vi "Main.vi"(11 "Module Admin":refnum<class "Delacor_lib_QMH_Cloneable Module Admin.lvclass">) -> ()   [LabVIEW 2020, in "Cloneable Module.lvlib"]
doc: "This template is based off of the Queued Message Handler design pattern and the Queued Message Handler project template that ships with LabVIEW.\n\nThe main difference is that the queue is private to this module and communication between modules is performed via Broadcast and Request events.\n\nRequest events are wrapped in public API methods and are handled in the Event Handling Loop (EHL) of this VI. Any module can register for Broadcast events sent by this module. The EHL generates messages based on user interface actions.\n\nThe Message Handling Loop (MHL) processes messages generated by the EHL, or by other messages. The messages are string values, so new messages can be added easily to the Message Cases case structure in the MHL. Each message cluster can also provide an optional value for Message Data, which is a variant that can be converted to whatever message-specific data is required.\n_____\nBased on DQMH Project Template 6.1.0.93."
uses:
  Cloneable Module.lvlib
  <vilib>/Delacor/Delacor QMH/Libraries/Message Queue_class/Delacor_lib_QMH_Message Queue.lvclass
  Module Data--cluster.ctl
  <vilib>/Utility/miscctls.llb/LVPointTypeDef.ctl
  Do Something Argument--cluster.ctl
  Do Something Else Argument--cluster.ctl
  Do Something Else and Wait (Reply Payload)--cluster.ctl
  Do Something Else and Wait for Reply Argument--cluster.ctl
  <vilib>/Utility/error.llb/Error Cluster From Error Code.vi
  <vilib>/ErrorRing/Error Ring.xnode
  <vilib>/Delacor/Delacor QMH/Libraries/Message Queue_class/Delacor_lib_QMH_Enqueue Message (Single).vi
  Stop Argument--cluster.ctl
  <vilib>/Delacor/Delacor QMH/Libraries/Cloneable Module Admin_class/Delacor_lib_QMH_Cloneable Module Admin.lvclass
  ADD (Reply Payload)--cluster.ctl
  ADD Argument--cluster.ctl
panel:
  out "error out":errorcluster
  out "X":dbl
  out "Status":string
  in  "Simulate EHL Error":bool
  in  "Simulate MHL Error":bool
  in  "Do Something Else <Replace Me>":bool
  in  "Do Something <Replace Me>":bool
  # "These controls have associated \"Value Changed\" events configured in the Event Structure on the diagram.\n\nReplace them (and reconfigure the Event Structure) with the controls you need for your application. \n\nOther QMH Modules communicate with this Module via its Public API (wrappers for its Request Events).\n\nThis Module communicates with other Modules via its Broadcast Events.\nAny module that wants to get these messages, just registers for this module's Broadcast events."
  # "This template is for the Delacor Modified Queued Message Handler design pattern.\n\nSee the block diagram for more information on how to use this template."
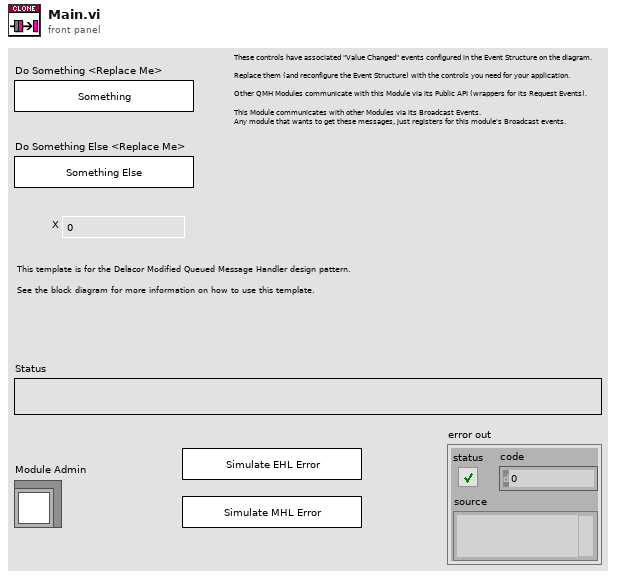
[diagram p1: front panel]
types:
  T1 = typedef "Cloneable Module.lvlib/Request Events--cluster.ctl" = cluster{"Stop Module":refnum<user-event>, "Do Something":refnum<user-event>, "Do Something Else":refnum<user-event>, "Do Something Else and Wait for Reply":refnum<user-event>, "Show Panel":refnum<user-event>, "Hide Panel":refnum<user-event>, "Show Diagram":refnum<user-event>, "Get Module Execution Status":refnum<user-event>, "ADD":refnum<user-event>}
  T2 = typedef "Cloneable Module.lvlib/Module Data--cluster.ctl" = cluster{"Status":string}
  T3 = typedef "Cloneable Module.lvlib/Do Something Argument--cluster.ctl" = cluster{"Module ID":i32, "Do Something Msg":string}
  T4 = typedef "Cloneable Module.lvlib/Do Something Else Argument--cluster.ctl" = cluster{"Module ID":i32, "Do Something Else Msg":string, "X":dbl}
  T5 = typedef "Cloneable Module.lvlib/Do Something Else and Wait for Reply Argument--cluster.ctl" = cluster{"Module ID":i32, "Do Something Else Msg":string, "X":dbl, "Wait Notifier":refnum<notifier>, "wait for reply":bool}
  T6 = enum32{"invalid lock state", "Not Locked", "Locked (No Password)", "Password-protected"}
  T7 = typedef "Cloneable Module.lvlib/Stop Argument--cluster.ctl" = cluster{"Module ID":i32, "Origin":string, "Exit via Stop Module Req?":bool, "Wait for Module to stop?":bool}
  T8 = typedef "Cloneable Module.lvlib/ADD Argument--cluster.ctl" = cluster{"Module ID":i32, "A":dbl, "B":dbl, "Wait Notifier":refnum<notifier>, "wait for reply":bool}
  T9 = typedef "LVPointTypeDef.ctl" = cluster{"Horizontal":i16, "Vertical":i16}
  T10 = enum32{"Invalid", "Standard", "Closed", "Hidden", "Minimized", "Maximized"}
  T11 = typedef "Cloneable Module.lvlib/Do Something Else and Wait (Reply Payload)--cluster.ctl" = cluster{"Value":dbl, "error":errorcluster}
  T12 = typedef "Cloneable Module.lvlib/ADD (Reply Payload)--cluster.ctl" = cluster{"A+B":dbl, "error":errorcluster}
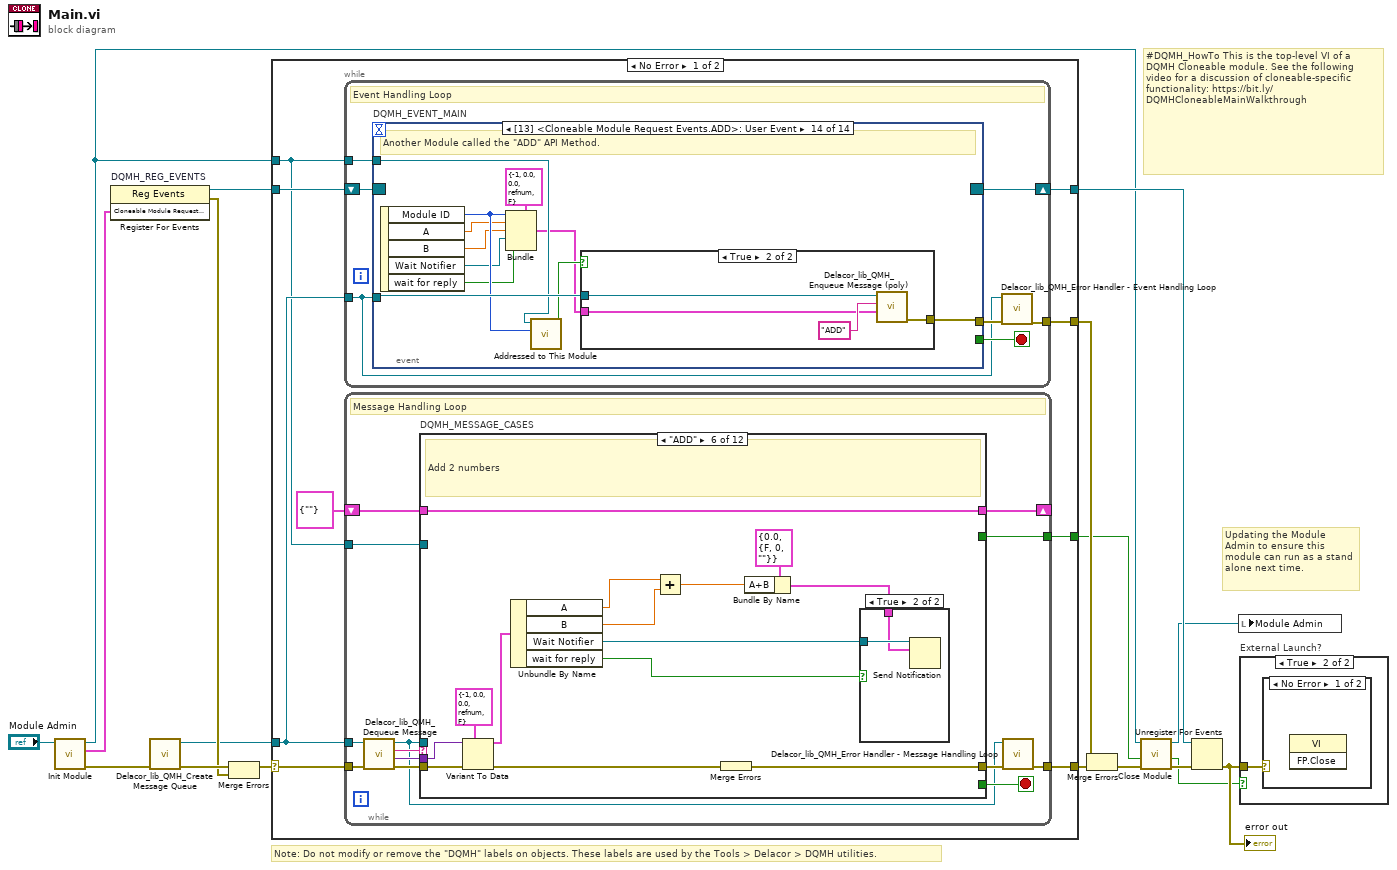
[diagram p0: block diagram]
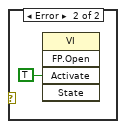
[diagram p3: hidden frame]
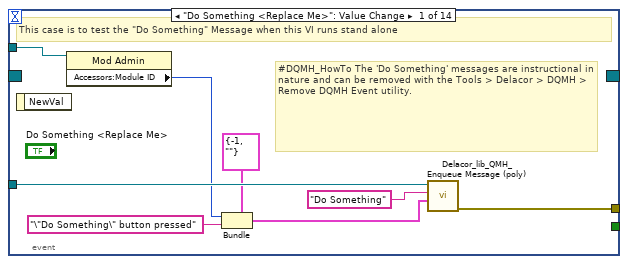
[diagram p4: hidden frame]
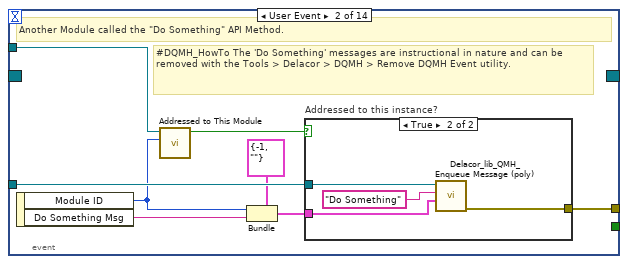
[diagram p5: hidden frame]
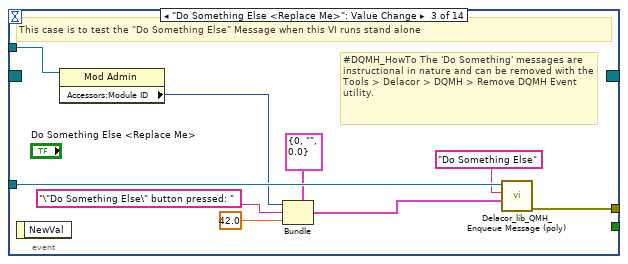
[diagram p7: hidden frame]
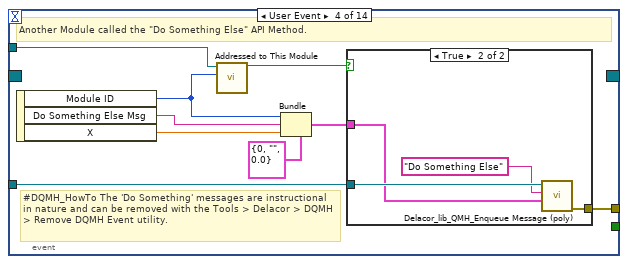
[diagram p8: hidden frame]
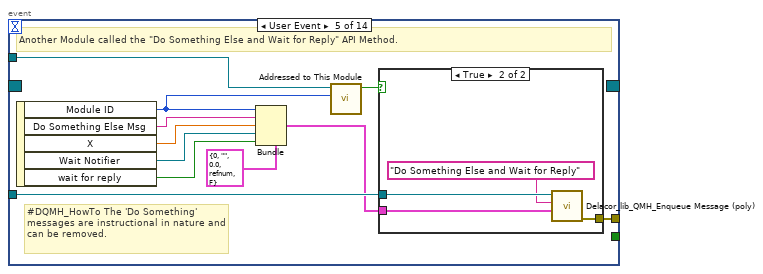
[diagram p10: hidden frame]
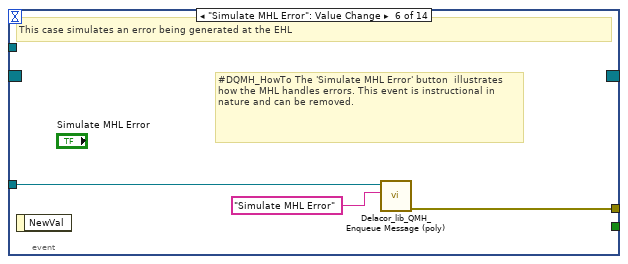
[diagram p12: hidden frame]
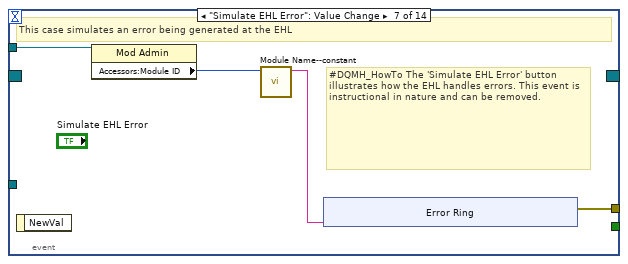
[diagram p13: hidden frame]
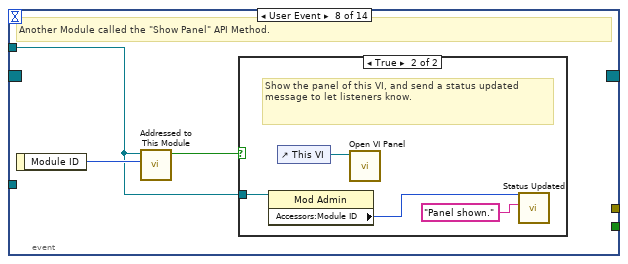
[diagram p14: hidden frame]
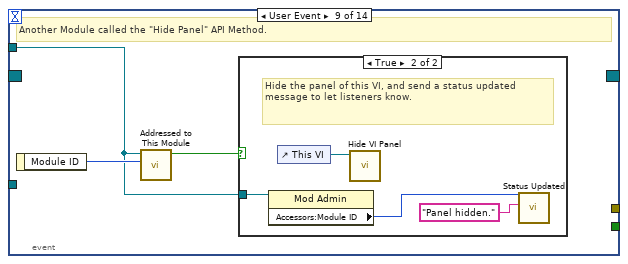
[diagram p16: hidden frame]
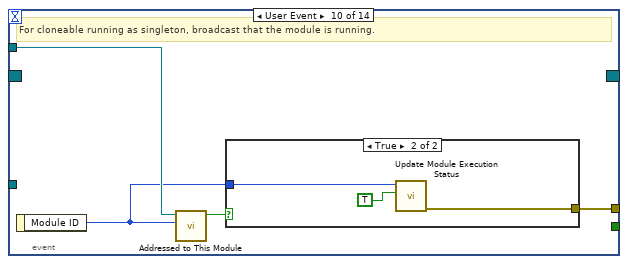
[diagram p18: hidden frame]
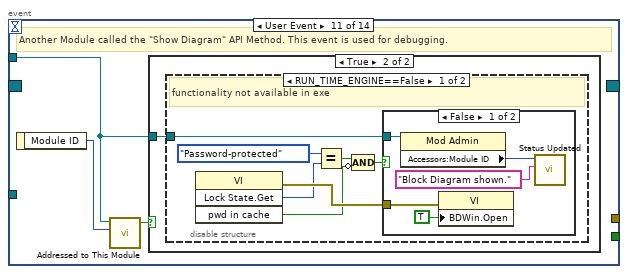
[diagram p20: hidden frame]
diagram:
  # "#DQMH_HowTo This is the top-level VI of a DQMH Cloneable module. See the following video for a discussion of cloneable-specific functionality: https://bit.ly/DQMHCloneableMainWalkthrough"
  # "Note: Do not modify or remove the \"DQMH\" labels on objects. These labels are used by the Tools > Delacor > DQMH utilities."
  # "Updating the Module Admin to ensure this module can run as a stand alone next time."
  n1 = call "Init Module.vi"("Cloneable Module Admin in"="Module Admin") -> ("error out"=w15:errorcluster, "Cloneable Module Request Events"=w7:T1, "Cloneable Module Admin out"=w4:refnum<class "Delacor_lib_QMH_Cloneable Module Admin.lvclass">)  [unwired: 8 in]
  n2 = register-events "DQMH_REG_EVENTS"(w7) -> (reference out=w8:refnum<event-registration>, error out=w10:errorcluster)  [unwired: 2 in]
  n3 = call <vilib>:"Delacor_lib_QMH_Create Message Queue.vi"("error in"=w15) -> ("error out"=w12:errorcluster, "Message Queue"=w6:refnum<class "Delacor_lib_QMH_Message Queue.lvclass">)  [unwired: 9 in]
  n4 = Merge Errors(w12, w10) -> (w11:errorcluster)
  n5 = case shown="No Error" w11 {
    selector: w11 -> [w25 w365]
    tunnel: [w27 w364] -> w16
    tunnel: [w24 w372] -> w9
    tunnel: w8 -> [w22 w372]
    tunnel: w6 -> [w21 w363]
    tunnel: [w26 _] -> w17
    tunnel: w4 -> [w20 w368]
    tunnel: [w19 _] -> w2
    frame No Error {
      n6 = while {
        tunnel: w21 -> [w28]
        shift-right: [w31] -> w24
        shift-left: w22 -> [w32]
        tunnel: [w33] -> w26
        tunnel: w20 -> [w29]
        stop <- w30 stop-if-true
        # "Event Handling Loop"
        n7 = event "DQMH_EVENT_MAIN" shown="[13] <Cloneable Module Request Events.ADD>: User Event" {
          selector: w32 -> [_ _ _ _ _ _ _ _ _ _ _ _ _ _]
          dyn-events: [_ _ _ _ _ _ _ _ _ _ _ _ _ _] -> w31
          timeout: _ -> [_ _ _ _ _ _ _ _ _ _ _ _ _ _]
          tunnel: [_ _ _ _ _ _ _ _ _ _ _ w146 _ _] -> w30
          tunnel: w28 -> [w41 w49 w62 w71 w86 w93 _ _ _ _ _ w149 w165 w184]
          tunnel: [w42 w50 w63 w72 w87 w94 w98 _ _ w123 _ w150 w168 w174] -> w34
          tunnel: w29 -> [w37 w47 w56 w69 w84 _ w97 w106 w113 w121 w127 w148 w166 w182]
          event "Do Something <Replace Me>": Value Change {
            # "#DQMH_HowTo The 'Do Something' messages are instructional in nature and can be removed with the Tools > Delacor > DQMH > Remove DQMH Event utility."
            # "This case is to test the \"Do Something\" Message when this VI runs stand alone"
            n8 = event-data() -> ()  [unwired: 1 in, 1 out]
            n9 = property class="Mod Admin"(reference=w37) -> ("Accessors:Module ID"=w36:i32)  [unwired: 1 in, 2 out]
            n10 = Bundle(cluster=T3 {"Module ID"=-1, "Do Something Msg"=""} ("Do Something Argument"), "Module ID"=w36, "Do Something Msg"="\"Do Something\" button pressed" ("\"Do Something\" button pressed")) -> (w39:T3)
            n11 = call-poly <vilib>:"Delacor_lib_QMH_Enqueue Message (poly).vi"("Message Data"=w39, "Message"="Do Something", "Message Queue in"=w41) -> ("error out"=w42:errorcluster)  [unwired: 7 in, 1 out]
          }
          event User Event {
            # "#DQMH_HowTo The 'Do Something' messages are instructional in nature and can be removed with the Tools > Delacor > DQMH > Remove DQMH Event utility."
            # "Another Module called the \"Do Something\" API Method."
            n12 = event-data() -> ("Module ID"=w44:i32, "Do Something Msg"=w43:string)  [unwired: 1 in]
            n13 = call "Addressed to This Module.vi"("Module ID from Argument"=w44, "Module Admin"=w47) -> ("Addressed to this instance?"=w48:bool)  [unwired: 8 in, 1 out]
            n14 = Bundle(cluster=T3 {"Module ID"=-1, "Do Something Msg"=""} ("Do Something Argument"), "Module ID"=w44, "Do Something Msg"=w43) -> (w46:T3)
            n15 = case "Addressed to this instance?" shown="True" w48 {
              tunnel: w49 -> [_ w53]
              tunnel: [_ w54] -> w50
              tunnel: w46 -> [_ w51]
              frame False {
                # "Do nothing"
              }
              frame True {
                n16 = call-poly <vilib>:"Delacor_lib_QMH_Enqueue Message (poly).vi"("Message Data"=w51, "Message"="Do Something", "Message Queue in"=w53) -> ("error out"=w54:errorcluster)  [unwired: 7 in, 1 out]
              }
            }
          }
          event "Do Something Else <Replace Me>": Value Change {
            # "#DQMH_HowTo The 'Do Something' messages are instructional in nature and can be removed with the Tools > Delacor > DQMH > Remove DQMH Event utility."
            # "This case is to test the \"Do Something Else\" Message when this VI runs stand alone"
            n17 = event-data() -> ()  [unwired: 1 in, 1 out]
            n18 = property class="Mod Admin"(reference=w56) -> ("Accessors:Module ID"=w55:i32)  [unwired: 1 in, 2 out]
            n19 = Bundle(cluster=T4 {"Module ID"=0, "Do Something Else Msg"="", "X"=0.0} ("Do Something Else Argument"), "Module ID"=w55, "Do Something Else Msg"="\"Do Something Else\" button pressed: " ("\"Do Something Else\" button pressed"), "X"=42.0) -> (w59:T4)
            n20 = call-poly <vilib>:"Delacor_lib_QMH_Enqueue Message (poly).vi"("Message Data"=w59, "Message"="Do Something Else", "Message Queue in"=w62) -> ("error out"=w63:errorcluster)  [unwired: 7 in, 1 out]
          }
          event User Event {
            # "#DQMH_HowTo The 'Do Something' messages are instructional in nature and can be removed with the Tools > Delacor > DQMH > Remove DQMH Event utility."
            # "Another Module called the \"Do Something Else\" API Method."
            n21 = event-data() -> ("Module ID"=w64:i32, "Do Something Else Msg"=w65:string, "X"=w67:dbl)  [unwired: 1 in]
            n22 = call "Addressed to This Module.vi"("Module ID from Argument"=w64, "Module Admin"=w69) -> ("Addressed to this instance?"=w70:bool)  [unwired: 8 in, 1 out]
            n23 = Bundle(cluster=T4 {"Module ID"=0, "Do Something Else Msg"="", "X"=0.0} ("Do Something Else Argument"), "Module ID"=w64, "Do Something Else Msg"=w65, "X"=w67) -> (w66:T4)
            n24 = case shown="True" w70 {
              tunnel: w71 -> [_ w75]
              tunnel: [_ w76] -> w72
              tunnel: w66 -> [_ w73]
              frame False {
              }
              frame True {
                n25 = call-poly <vilib>:"Delacor_lib_QMH_Enqueue Message (poly).vi"("Message Data"=w73, "Message"="Do Something Else", "Message Queue in"=w75) -> ("error out"=w76:errorcluster)  [unwired: 7 in, 1 out]
              }
            }
          }
          event User Event {
            # "#DQMH_HowTo The 'Do Something' messages are instructional in nature and can be removed."
            # "Another Module called the \"Do Something Else and Wait for Reply\" API Method."
            n26 = event-data() -> ("Module ID"=w82:i32, "Do Something Else Msg"=w80:string, "X"=w79:dbl, "Wait Notifier"=w78:refnum<notifier>, "wait for reply"=w77:bool)  [unwired: 1 in]
            n27 = Bundle(cluster=T5 {"Module ID"=0, "Do Something Else Msg"="", "X"=0.0, "Wait Notifier"=refnum, "wait for reply"=FALSE} ("Do Something Else and Wait for Reply Argument"), "Module ID"=w82, "Do Something Else Msg"=w80, "X"=w79, "Wait Notifier"=w78, "wait for reply"=w77) -> (w81:T5)
            n28 = call "Addressed to This Module.vi"("Module ID from Argument"=w82, "Module Admin"=w84) -> ("Addressed to this instance?"=w85:bool)  [unwired: 8 in, 1 out]
            n29 = case shown="True" w85 {
              tunnel: [_ w91] -> w87
              tunnel: w86 -> [_ w90]
              tunnel: w81 -> [_ w88]
              frame False {
              }
              frame True {
                n30 = call-poly <vilib>:"Delacor_lib_QMH_Enqueue Message (poly).vi"("Message Data"=w88, "Message"="Do Something Else and Wait for Reply", "Message Queue in"=w90) -> ("error out"=w91:errorcluster)  [unwired: 7 in, 1 out]
              }
            }
          }
          event "Simulate MHL Error": Value Change {
            # "#DQMH_HowTo The 'Simulate MHL Error' button  illustrates how the MHL handles errors. This event is instructional in nature and can be removed."
            # "This case simulates an error being generated at the EHL"
            n31 = event-data() -> ()  [unwired: 1 in, 1 out]
            n32 = call-poly <vilib>:"Delacor_lib_QMH_Enqueue Message (poly).vi"("Message"="Simulate MHL Error", "Message Queue in"=w93) -> ("error out"=w94:errorcluster)  [unwired: 8 in, 1 out]
          }
          event "Simulate EHL Error": Value Change {
            # "#DQMH_HowTo The 'Simulate EHL Error' button  illustrates how the EHL handles errors. This event is instructional in nature and can be removed."
            # "This case simulates an error being generated at the EHL"
            n33 = event-data() -> ()  [unwired: 1 in, 1 out]
            n34 = property class="Mod Admin"(reference=w97) -> ("Accessors:Module ID"=w96:i32)  [unwired: 1 in, 2 out]
            n35 = call "Module Name--constant.vi"("Module ID"=w96) -> ("Module Name"=w95:string)  [unwired: 10 in]
            n36 = xnode "Error Ring"("parameter 0"=w95) -> ("error out"=w98:errorcluster)
          }
          event User Event {
            # "Another Module called the \"Show Panel\" API Method."
            n37 = event-data() -> ("Module ID"=w107:i32)  [unwired: 1 in]
            n38 = call "Addressed to This Module.vi"("Module ID from Argument"=w107, "Module Admin"=w106) -> ("Addressed to this instance?"=w108:bool)  [unwired: 8 in, 1 out]
            n39 = case shown="True" w108 {
              tunnel: w106 -> [_ w110]
              frame False {
              }
              frame True {
                # "Show the panel of this VI, and send a status updated message to let listeners know."
                n40 = property class="Mod Admin"(reference=w110) -> ("Accessors:Module ID"=w109:i32)  [unwired: 1 in, 2 out]
                n41 = control-ref of="This VI"() -> (w112:refnum<vi>)
                n42 = call "Open VI Panel.vi"("VI"=w112) -> ()  [unwired: 10 in, 1 out]
                n43 = call "Status Updated.vi"("Status"="Panel shown." ("format string"), "Module ID"=w109) -> ()  [unwired: 9 in, 1 out]
              }
            }
          }
          event User Event {
            # "Another Module called the \"Hide Panel\" API Method."
            n44 = event-data() -> ("Module ID"=w114:i32)  [unwired: 1 in]
            n45 = call "Addressed to This Module.vi"("Module ID from Argument"=w114, "Module Admin"=w113) -> ("Addressed to this instance?"=w115:bool)  [unwired: 8 in, 1 out]
            n46 = case shown="True" w115 {
              tunnel: w113 -> [_ w117]
              frame False {
              }
              frame True {
                # "Hide the panel of this VI, and send a status updated message to let listeners know."
                n47 = property class="Mod Admin"(reference=w117) -> ("Accessors:Module ID"=w116:i32)  [unwired: 1 in, 2 out]
                n48 = control-ref of="This VI"() -> (w119:refnum<vi>)
                n49 = call "Hide VI Panel.vi"("VI"=w119) -> ()  [unwired: 10 in, 1 out]
                n50 = call "Status Updated.vi"("Status"="Panel hidden." ("format string"), "Module ID"=w116) -> ()  [unwired: 9 in, 1 out]
              }
            }
          }
          event User Event {
            # "For cloneable running as singleton, broadcast that the module is running."
            n51 = event-data() -> ("Module ID"=w120:i32)  [unwired: 1 in]
            n52 = call "Addressed to This Module.vi"("Module ID from Argument"=w120, "Module Admin"=w121) -> ("Addressed to this instance?"=w122:bool)  [unwired: 8 in, 1 out]
            n53 = case shown="True" w122 {
              tunnel: [_ w126] -> w123
              tunnel: w120 -> [_ w125]
              frame False {
              }
              frame True {
                n54 = call "Update Module Execution Status.vi"("Running?"=TRUE, "Module ID"=w125) -> ("error out"=w126:errorcluster)  [unwired: 9 in]
              }
            }
          }
          event User Event {
            # "Another Module called the \"Show Diagram\" API Method. This event is used for debugging."
            n55 = event-data() -> ("Module ID"=w128:i32)  [unwired: 1 in]
            n56 = call "Addressed to This Module.vi"("Module ID from Argument"=w128, "Module Admin"=w127) -> ("Addressed to this instance?"=w129:bool)  [unwired: 8 in, 1 out]
            n57 = case shown="True" w129 {
              tunnel: w127 -> [_ w130]
              frame False {
              }
              frame True {
                n58 = disable-structure shown="RUN_TIME_ENGINE==False" {
                  disable-tunnel: w130 -> [w131 _]
                  frame condition #0 (active) {
                    # "functionality not available in exe"
                    n59 = invoke class="VI" method="Lock State.Get"() -> (error out=w137:errorcluster, "Get Lock State"=w136:T6, "pwd in cache"=w133:bool)  [unwired: 4 in, 1 out]
                    n60 = Equal?(x=T6."Password-protected", y=w136) -> (x = y?=w134:bool)
                    n61 = Compound Arithmetic op=AND(w134, invert w133) -> (w132:bool)
                    n62 = case shown="False" w132 {
                      tunnel: w137 -> [w142 _]
                      tunnel: w131 -> [w139 _]
                      frame False {
                        n63 = property class="Mod Admin"(reference=w139) -> ("Accessors:Module ID"=w138:i32)  [unwired: 1 in, 2 out]
                        n64 = property class="VI"(error in=w142, "BDWin.Open"=TRUE ("Block Diagram Window:Open")) -> ()  [unwired: 1 in, 2 out]
                        n65 = call "Status Updated.vi"("Status"="Block Diagram shown." ("format string"), "Module ID"=w138) -> ()  [unwired: 9 in, 1 out]
                      }
                      frame True {
                        # "Password-protected VI, and the password is not in the cache. Do not show the diagram."
                      }
                    }
                  }
                  frame condition #1 {
                  }
                }
              }
            }
          }
          event User Event {
            # "Another Module called the \"Stop Module\" API Method  or the Message Handling Loop below."
            n66 = event-data() -> ("Module ID"=w144:i32, "Wait for Module to stop?"=w145:bool, "Origin"=w143:string)  [unwired: 1 in]
            n67 = call "Addressed to This Module.vi"("Module ID from Argument"=w144, "Module Admin"=w148) -> ("Addressed to this instance?"=w147:bool)  [unwired: 8 in, 1 out]
            n68 = case shown="True" w147 {
              tunnel: [_ w162] -> w150
              tunnel: w149 -> [_ w158]
              tunnel: [_ TRUE] -> w146
              tunnel: w145 -> [_ w153]
              tunnel: w144 -> [_ w155]
              tunnel: w143 -> [_ w151]
              frame False {
              }
              frame True {
                # "The event can get fired from the Exit message. The queue gets destroyed there. In this case, the Enqueue VI will return error 1. It is safe to ignore, because the module is already exiting."
                n69 = local write "Status"(w151) -> ()
                n70 = Bundle By Name(cluster=T7 {"Module ID"=-1, "Origin"="", "Exit via Stop Module Req?"=FALSE, "Wait for Module to stop?"=FALSE} ("Stop Argument"), "Module ID"=w155, "Exit via Stop Module Req?"=TRUE, "Wait for Module to stop?"=w153) -> (w152:T7)
                n71 = call-poly <vilib>:"Delacor_lib_QMH_Enqueue Message (poly).vi"("Priority Message? (F)"=TRUE, "Message Data"=w152, "Message"="Exit", "Message Queue in"=w158) -> ("error out"=w163:errorcluster)  [unwired: 6 in, 1 out]
                n72 = call <vilib>:"Clear Errors.vi"("error in (no error)"=w163, "specific error code to clear (0: all)"=1) -> ("error out"=w162:errorcluster)  [unwired: 4 in, 1 out]
              }
            }
          }
          event Panel Close? {
            w167 = TRUE  # Discard the event, the MHL is responsible for closing and stopping this VI.
            # "Hide the panel or send the 'Exit' message if the user clicks the 'X' on the module main VI panel."
            n73 = event-data() -> ()  [unwired: 1 in, 1 out]
            n74 = property class="Mod Admin"(reference=w166) -> ("Accessors:External Launch"=w164:bool)  [unwired: 1 in, 2 out]
            n75 = case shown="True" w164 {
              tunnel: w165 -> [_ w172]
              tunnel: [_ w173] -> w168
              frame True {
                # "If externally launched, clicking the 'X' hides the panel, but doesn't close it."
                n76 = control-ref of="This VI"() -> (w169:refnum<vi>)
                n77 = call "Hide VI Panel.vi"("VI"=w169) -> ()  [unwired: 10 in, 1 out]
              }
              frame False {
                # "If run as a stand-alone VI, clicking the panel 'X' stops the VI."
                n78 = call-poly <vilib>:"Delacor_lib_QMH_Enqueue Message (poly).vi"("Priority Message? (F)"=TRUE, "Message"="Exit", "Message Queue in"=w172) -> ("error out"=w173:errorcluster)  [unwired: 7 in, 1 out]
              }
            }
            n79 = event-data("Discard?"=w167) -> ()  [unwired: 1 in, 1 out]
          }
          event User Event {
            # "Another Module called the \"ADD\" API Method."
            n80 = event-data() -> ("Module ID"=w179:i32, "A"=w178:dbl, "B"=w177:dbl, "Wait Notifier"=w176:refnum<notifier>, "wait for reply"=w175:bool)  [unwired: 1 in]
            n81 = Bundle(cluster=T8 {"Module ID"=-1, "A"=0.0, "B"=0.0, "Wait Notifier"=refnum, "wait for reply"=FALSE} ("ADD Argument"), "Module ID"=w179, "A"=w178, "B"=w177, "Wait Notifier"=w176, "wait for reply"=w175) -> (w180:T8)
            n82 = call "Addressed to This Module.vi"("Module ID from Argument"=w179, "Module Admin"=w182) -> ("Addressed to this instance?"=w183:bool)  [unwired: 8 in, 1 out]
            n83 = case shown="True" w183 {
              tunnel: w184 -> [_ w188]
              tunnel: w180 -> [_ w186]
              tunnel: [_ w185] -> w174
              frame False {
              }
              frame True {
                n84 = call-poly <vilib>:"Delacor_lib_QMH_Enqueue Message (poly).vi"("Message Data"=w186, "Message"="ADD", "Message Queue in"=w188) -> ("error out"=w185:errorcluster)  [unwired: 7 in, 1 out]
              }
            }
          }
        }
        n85 = call-dynamic "Delacor_lib_QMH_Error Handler - Event Handling Loop.vi"("error in"=w34, "Message Queue in"=w28) -> ("dup error in"=w33:errorcluster)  [unwired: 8 in, 1 out]
      }
      n86 = while {
        tunnel: w21 -> [w192]
        shift-right: [w196] -> _
        shift-left: T2 {"Status"=""} ("Data Cluster") -> [w197]
        tunnel: w25 -> [w200]
        tunnel: [w198] -> w27
        tunnel: w20 -> [w190]
        tunnel: [w189] -> w19
        stop <- w195 stop-if-true
        # "Message Handling Loop"
        n87 = call-dynamic "Delacor_lib_QMH_Dequeue Message.vi"("error in"=w200, "Message Queue in"=w192) -> ("error out"=w199:errorcluster, "Message Data"=w193:variant, "Message"=w194:string, "Message Queue out"=w191:refnum<class "Delacor_lib_QMH_Message Queue.lvclass">)  [unwired: 6 in]
        n88 = case "DQMH_MESSAGE_CASES" shown="\"ADD\"" w194 {
          selector: w194 -> [_ _ _ _ _ _ _ _ _ _ _ w350]
          tunnel: w191 -> [_ _ _ _ _ _ _ _ w301 _ w340 _]
          tunnel: w199 -> [w220 w224 w234 w245 w266 w292 w297 w299 w310 w323 w346 w352]
          tunnel: [w218 w224 w232 w244 w265 w282 w296 w299 w306 w322 w343 w353] -> w201
          tunnel: w197 -> [w211 w223 w231 w243 w263 w291 w295 w298 w305 w320 w339 w351]
          tunnel: [w210 w223 w231 w243 w263 w291 w295 w298 w305 w320 w339 w351] -> w196
          tunnel: [_ _ _ _ _ _ _ _ _ _ w338 _] -> w195
          tunnel: w193 -> [_ _ w230 w240 w260 w289 _ _ w304 _ w336 _]
          tunnel: w190 -> [w205 _ w226 w236 w250 _ _ _ w303 w318 w332 w348]
          tunnel: [_ _ _ _ _ _ _ _ _ _ w334 _] -> w189
          frame "Initialize" {
            w202 = "Initial Message" ("Initial Message")
            # "#CodeNeeded - Initialize the appearance of the front panel."
            # "#CodeNeeded - Initialize your state data here."
            # "Initialize - Any operation that needs to be done before the module can receive messages. Synchronize Caller Events.vi will inform Start Module.vi that the module has launched and is ready to receive messages. Module Did Init.vi will broadcast that the module initialized."
            n89 = call "Synchronize Caller Events.vi"("error in (no error)"=w220, "Module Admin"=w205) -> ("error out"=w219:errorcluster, "Module Admin out"=w204:refnum<class "Delacor_lib_QMH_Cloneable Module Admin.lvclass">)  [unwired: 8 in]
            n90 = property class="Mod Admin"(reference=w204) -> ("Accessors:Module ID"=w207:i32, "Accessors:External Launch"=w206:bool)  [unwired: 1 in, 2 out]
            n91 = call "Module Name--constant.vi"("Module ID"=w207) -> ("Module Name"=w215:string)  [unwired: 10 in]
            n92 = property class="VI"("Front Panel.Title"=w215) -> (reference out=w217:refnum<vi>, error out=w222:errorcluster)  [unwired: 2 in]
            n93 = Select(t=T10."Hidden" ("State"), s=w206, f=T10."Standard" ("State")) -> (s? t:f=w212:T10)
            n94 = invoke class="VI" method="FP.Open"(reference=w217, error in=w222, "State"=w212) -> (reference out=w216:refnum<vi>, error out=w221:errorcluster)  [unwired: 2 in, 3 out]
            n95 = call "Module Name--constant.vi"("Module ID"=w207) -> ("Module Name"=w208:string)  [unwired: 10 in]
            n96 = Bundle By Name(cluster=w211, "Status"=w202) -> (w210:T2)
            n97 = invoke class="VI" method="FP.Center"(reference=w216, error in=w221) -> ()  [unwired: 1 in, 3 out]
            n98 = property on="Pane" class="Pane"("Origin"=T9 {"Horizontal"=0, "Vertical"=0}) -> ()  [unwired: 2 in, 2 out]
            n99 = call "Module Did Init.vi"("error in (no error)"=w219, "Initialized?"=TRUE, "Origin"=w208, "Module ID"=w207) -> ("error out"=w218:errorcluster)  [unwired: 7 in]
            "Status" <- w202
          }
          frame "---Module Specific---" {
            # "Separator -- The following cases handle messages specific to this Module."
          }
          frame "Do Something" {
            # "#DQMH_HowTo The 'Do Something' messages are instructional in nature and can be removed with the Tools > Delacor > DQMH > Remove DQMH Event utility."
            # "Do Something - Replace this message with functionality for your own application. Note that this message also fires the \"Did Something\" broadcast event."
            n100 = property class="Mod Admin"(reference=w226) -> ("Accessors:Module ID"=w225:i32)  [unwired: 1 in, 2 out]
            n101 = Variant To Data(error in=w234, type=T3 {"Module ID"=-1, "Do Something Msg"=""} ("Do Something Argument"), Variant=w230) -> (data=w229:T3, error out=w233:errorcluster)
            n102 = Unbundle By Name(w229) -> ("Do Something Msg"=w227:string)
            n103 = call "Status Updated.vi"("Status"=w227, "Module ID"=w225) -> ()  [unwired: 9 in, 1 out]
            n104 = local write "Status"(w227) -> ()
            n105 = call "Did Something.vi"("error in (no error)"=w233, "Did Something Msg"=w227, "Module ID"=w225) -> ("error out"=w232:errorcluster)  [unwired: 8 in]
          }
          frame "Do Something Else" {
            # "#DQMH_HowTo The 'Do Something' messages are instructional in nature and can be removed with the Tools > Delacor > DQMH > Remove DQMH Event utility."
            # "Do Something Else - Replace this message with functionality for your own application."
            n106 = Variant To Data(error in=w245, type=T4 {"Module ID"=0, "Do Something Else Msg"="", "X"=0.0} ("Do Something Else Argument"), Variant=w240) -> (data=w241:T4, error out=w244:errorcluster)
            n107 = Unbundle By Name(w241) -> ("Do Something Else Msg"=w239:string, "X"=w238:dbl)
            "X" <- w238
            n108 = property class="Mod Admin"(reference=w236) -> ("Accessors:Module ID"=w235:i32)  [unwired: 1 in, 2 out]
            n109 = Format Into String(initial string=w239, w238) -> (resulting string=w237:string)  [unwired: 2 in, 1 out]
            n110 = call "Status Updated.vi"("Status"=w237, "Module ID"=w235) -> ()  [unwired: 9 in, 1 out]
            n111 = local write "Status"(w237) -> ()
          }
          frame "Do Something Else and Wait for Reply" {
            w253 = "X(%.2f)+Offset(%.2f)=%.2f"  # status message format string
            # "#DQMH_HowTo The 'Do Something' messages are instructional in nature and can be removed."
            # "Send back X with a random offset"
            # "Do Something Else and Wait for Reply - Replace this message with functionality for your own application. Note that this message must fire a notifier to let callers know it has finished execution, and it returns an error if the 'Value' is negative."
            n112 = Variant To Data(error in=w266, type=T5 {"Module ID"=0, "Do Something Else Msg"="", "X"=0.0, "Wait Notifier"=refnum, "wait for reply"=FALSE} ("Do Something Else and Wait for Reply Argument"), Variant=w260) -> (data=w261:T5, error out=w247:errorcluster)
            n113 = Unbundle By Name(w261) -> ("Wait Notifier"=w258:refnum<notifier>, "Do Something Else Msg"=w259:string, "X"=w255:dbl, "wait for reply"=w246:bool)
            n114 = property class="Mod Admin"(reference=w250) -> ("Accessors:Module ID"=w249:i32)  [unwired: 1 in, 2 out]
            n115 = Random Number (0-1)() -> (number: 0 to 1=w254:dbl)
            n116 = local write "X"(w255) -> ()
            n117 = Add(x=w254, y=w255) -> (x+y=w248:dbl)
            n118 = Format Into String(format string=w253, initial string=w259, w255, w254, w248) -> (resulting string=w251:string)  [unwired: 1 in, 1 out]
            n119 = Less Than 0?(x=w248) -> (x < 0?=w252:bool)
            n120 = case shown="True" w252 {
              tunnel: [_ w273] -> w264
              frame False {
              }
              frame True {
                n121 = xnode "Error Ring"() -> ("error out"=w273:errorcluster)
              }
            }
            n122 = Bundle By Name(cluster=T11 {"Value"=0.0, "error"={"status"=FALSE, "code"=0, "source"=""}} ("notification"), "error"=w264, "Value"=w248) -> (w256:T11)
            n123 = local write "Status"(w251) -> ()
            n124 = call "Status Updated.vi"("Status"=w251, "Module ID"=w249) -> ()  [unwired: 9 in, 1 out]
            n125 = case shown="True" w246 {
              tunnel: w258 -> [_ w270]
              tunnel: w256 -> [_ w269]
              frame False {
              }
              frame True {
                # "Simulate an operation that requires a wait."
                n126 = Wait (ms)(milliseconds to wait=u32 1000) -> (millisecond timer value=w267:u32)
                n127 = flat-sequence {
                  tunnel: w270 -> [w272]
                  tunnel: w269 -> [w271]
                  tunnel: w267 -> [_]
                  frame #0 {
                    n128 = Send Notification(notification=w271, notifier=w272) -> ()  [unwired: 1 in, 2 out]
                  }
                }
              }
            }
            n129 = Merge Errors(w247, w264) -> (w265:errorcluster)
          }
          frame "ADD" {
            # "Add 2 numbers"
            n130 = Variant To Data(error in=w292, type=T8 {"Module ID"=-1, "A"=0.0, "B"=0.0, "Wait Notifier"=refnum, "wait for reply"=FALSE} ("ADD Argument"), Variant=w289) -> (data=w287:T8, error out=w290:errorcluster)
            n131 = Unbundle By Name(w287) -> ("A"=w280:dbl, "B"=w279:dbl, "Wait Notifier"=w286:refnum<notifier>, "wait for reply"=w285:bool)
            n132 = Add(x=w280, y=w279) -> (x+y=w281:dbl)
            n133 = Merge Errors(w290) -> (w282:errorcluster)
            n134 = Bundle By Name(cluster=T12 {"A+B"=0.0, "error"={"status"=FALSE, "code"=0, "source"=""}} ("ADD (Reply Payload)"), "A+B"=w281) -> (w284:T12)
            n135 = case shown="True" w285 {
              tunnel: w286 -> [_ w294]
              tunnel: w284 -> [_ w293]
              frame False {
              }
              frame True {
                n136 = Send Notification(notification=w293, notifier=w294) -> ()  [unwired: 1 in, 2 out]
              }
            }
          }
          frame "---Copy This Frame---" {
            # "Duplicate this frame when creating new messages.  Change this comment in the duplicated frame to describe this message."
            n137 = Merge Errors(w297) -> (w296:errorcluster)
          }
          frame "---Exit and Error Handling---" {
            # "Separator - the following cases handle errors and exit messages."
          }
          frame "Error" {
            # "#CodeRecommended - If you ever change the name of this \"Error\" message, you'll need to update the name in the Check Loop Error.vi as well."
            # "#CodeRecommended - If the module is running in standalone mode (External Launch = FALSE), this code will pop up an error dialog and call the 'Exit' message if an error occurs. Add more fine-grained error handling here."
            # "Error - Check the error message data and respond accordingly. This message is sent by the \"Error Handler\" VIs at the end of each loop in this application."
            n138 = property class="Mod Admin"(reference=w303) -> ("Accessors:External Launch"=w302:bool, "Accessors:Module ID"=w300:i32)  [unwired: 1 in, 2 out]
            n139 = Variant To Data(error in=w310, type=errorcluster {"status"=FALSE, "code"=0, "source"=""} ("error constant"), Variant=w304) -> (data=w311:errorcluster, error out=w308:errorcluster)
            n140 = call "Error Reported.vi"("Error"=w311, "Module ID"=w300) -> ()  [unwired: 9 in, 1 out]
            n141 = case shown="False" w302 {
              tunnel: [w316 _] -> w307
              tunnel: w301 -> [w314 _]
              tunnel: w311 -> [w315 _]
              frame False {
                # "If the module is running standalone, then pop up an error dialog and call the \"Exit\" message."
                n142 = call <vilib>:"Simple Error Handler.vi"("error in (no error)"=w315) -> ()  [unwired: 4 in, 5 out]
                n143 = call-poly <vilib>:"Delacor_lib_QMH_Enqueue Message (poly).vi"("Priority Message? (F)"=TRUE, "Message"="Exit", "Message Queue in"=w314) -> ("error out"=w316:errorcluster)  [unwired: 7 in, 1 out]
              }
              frame True {
                # "If the module was launched externally, calling the Error Reported broadcast VI is the only action performed by the \"Error\" message. The module's caller can then process the error appropriately."
              }
            }
            n144 = Merge Errors(w308, w307) -> (w306:errorcluster)
            n145 = local write "error out"(w306) -> ()
          }
          frame "Simulate MHL Error" {
            # "#DQMH_HowTo The 'Simulate MHL Error' button  illustrates how the MHL handles errors. This event is instructional in nature and can be removed."
            # "Simulate an error occurring at the MHL"
            n146 = property class="Mod Admin"(reference=w318) -> ("Accessors:Module ID"=w319:i32)  [unwired: 1 in, 2 out]
            n147 = call "Module Name--constant.vi"("Module ID"=w319) -> ("Module Name"=w317:string)  [unwired: 10 in]
            n148 = xnode "Error Ring"("parameter 0"=w317) -> ("error out"=w321:errorcluster)
            n149 = Merge Errors(w323, w321) -> (w322:errorcluster)
          }
          frame "Exit" {
            w337 = 91  # 91: not all Exit messages will have an argument
            w338 = TRUE  # Stop the VI
            # "Release the message queue reference"
            # "#CodeNeeded - Add any required cleanup code here."
            # "Exit - Exit the application."
            n150 = Variant To Data(error in=w346, type=T7 {"Module ID"=-1, "Origin"="", "Exit via Stop Module Req?"=FALSE, "Wait for Module to stop?"=FALSE} ("Stop Argument"), Variant=w336) -> (data=w333:T7, error out=w341:errorcluster)
            n151 = call <vilib>:"Clear Errors.vi"("error in (no error)"=w341, "specific error code to clear (0: all)"=w337) -> ("error out"=w345:errorcluster)  [unwired: 4 in, 1 out]
            n152 = control-ref of="This VI"() -> (w331:refnum<vi>)
            n153 = call-dynamic "Delacor_lib_QMH_Release Message Queue.vi"("error in"=w345, "Message Queue"=w340) -> ("error out"=w344:errorcluster)  [unwired: 9 in]
            n154 = call "Handle Exit.vi"("Stop Argument"=w333, "Module Admin in"=w332, "VI reference"=w331) -> ("error out"=w342:errorcluster, "Wait for Stop?"=w334:bool)  [unwired: 7 in]
            n155 = Merge Errors(w344, w342) -> (w343:errorcluster)
          }
          frame Default {
            # "'Default' case only runs if there is a message that isn't defined in any of the other cases.  Output a programming error."
            n156 = property class="Mod Admin"(reference=w348) -> ("Accessors:Module ID"=w347:i32)  [unwired: 1 in, 2 out]
            n157 = call "Module Name--constant.vi"("Module ID"=w347) -> ("Module Name"=w349:string)  [unwired: 10 in]
            n158 = xnode "Error Ring"("parameter 0"=w350, "parameter 1"=w349) -> ("error out"=w354:errorcluster)
            n159 = Merge Errors(w352, w354) -> (w353:errorcluster)
          }
        }
        n160 = call-dynamic "Delacor_lib_QMH_Error Handler - Message Handling Loop.vi"("error in"=w201, "Message Queue in"=w191) -> ("dup error in"=w198:errorcluster)  [unwired: 8 in, 1 out]
      }
    }
    frame Error {
      n161 = call "Synchronize Caller Events.vi"("Module Admin"=w368) -> ("Module Admin out"=w367:refnum<class "Delacor_lib_QMH_Cloneable Module Admin.lvclass">)  [unwired: 9 in, 1 out]
      n162 = property class="Mod Admin"(reference=w367) -> ("Accessors:Module ID"=w366:i32)  [unwired: 1 in, 2 out]
      n163 = call-dynamic "Delacor_lib_QMH_Release Message Queue.vi"("error in"=w365, "Message Queue"=w363) -> ("error out"=w364:errorcluster)  [unwired: 9 in]
      n164 = call "Module Name--constant.vi"("Module ID"=w366) -> ("Module Name"=w371:string)  [unwired: 10 in]
      n165 = Format Into String(format string="An error occurred during initialization. %s is no longer running.", w371) -> (resulting string=w369:string)  [unwired: 2 in, 1 out]
      n166 = call "Error Reported.vi"("Additional Information"=w369, "Error"=w364, "Module ID"=w366) -> ()  [unwired: 8 in, 1 out]
    }
  }
  n167 = Merge Errors(w17, w16) -> (w18:errorcluster)
  n168 = call "Close Module.vi"("error in"=w18, "Wait for stop?"=w2, "Module Admin in"=w4) -> ("error out"=w14:errorcluster, "External Launch"=w1:bool, "Module Admin out"=w3:refnum<class "Delacor_lib_QMH_Cloneable Module Admin.lvclass">)  [unwired: 6 in]
  n169 = Unregister For Events(event registration refnum=w9, error in=w14) -> (error out=w13:errorcluster)
  "error out" <- w13
  n170 = local write "Module Admin"(w3) -> ()
  n171 = case "External Launch?" shown="True" w1 {
    tunnel: w13 -> [_ w373]
    frame False {
    }
    frame True {
      n172 = case shown="No Error" w373 {
        frame No Error {
          n173 = invoke class="VI" method="FP.Close"() -> ()  [unwired: 3 in, 3 out]
        }
        frame Error {
          n174 = invoke class="VI" method="FP.Open"("Activate"=TRUE ("Activate?")) -> ()  [unwired: 4 in, 5 out]
        }
      }
    }
  }
